vi "Take-Home-Ass.vi"() -> ()   [LabVIEW 2020]
panel:
  in  "Stop":bool
  in  "Thermometer":dbl(slide) scale=0.0..100.0
  in  "Take Measurement":bool
  out "Average Value":dbl
  out "Measurements":dbl[](array[numeric])
  out "Action":string
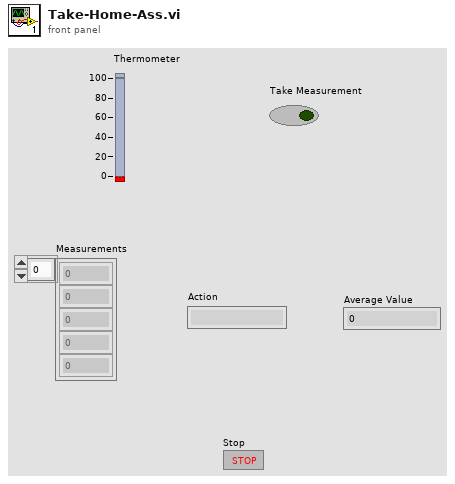
[diagram p1: front panel]
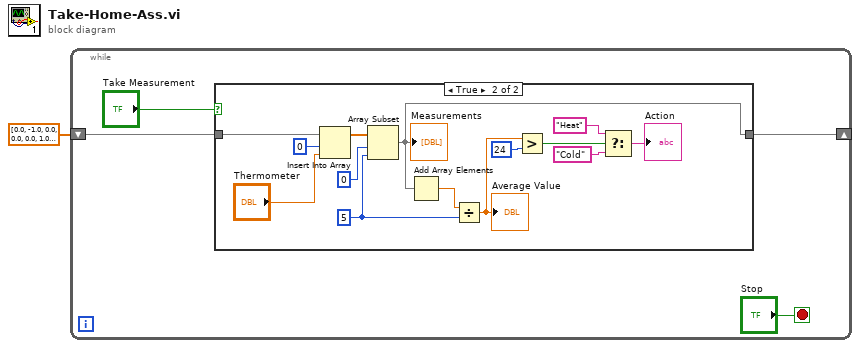
[diagram p0: block diagram]
diagram:
  n1 = while {
    shift-right: [w4] -> _
    shift-left: dbl[] [0.0, -1.0, 0.0, 0.0, 0.0, 1.0, 1.0, 2.0] ("Initial Array") -> [w5]
    stop <- "Stop" stop-if-true
    n2 = case shown="True" "Take Measurement" {
      tunnel: w5 -> [w6 w15]
      tunnel: [w6 w11] -> w4
      frame False {
      }
      frame True {
        w9 = 5
        n3 = Insert Into Array(array=w15, index=0, new element="Thermometer") -> (w13:dbl[])
        n4 = Array Subset(array=w13, index=0, length=w9) -> (w11:dbl[])
        "Measurements" <- w11
        n5 = Add Array Elements(numeric array=w11) -> (sum=w10:dbl)
        n6 = Divide(x=w10, y=w9) -> (x/y=w8:dbl)
        "Average Value" <- w8
        n7 = Greater?(x=w8, y=24) -> (0:w16:bool)
        n8 = Select(t="Heat", s=w16, f="Cold") -> (s? t:f=→"Action":string)
      }
    }
  }
